vi "Connect TCP.vi"(5 "Connection.TCP in":refnum<class "Connection.TCP.lvclass">, 6 "timeout (100ms)":i32=100, 8 "error in (no error)":errorcluster, 10 "remote port (80)":u16=80, 11 "address (localhost)":string="localhost") -> (0 "error out":errorcluster, 3 "Connection.TCP":refnum<class "Connection.TCP.lvclass">)   [LabVIEW 2013, in "Connection.TCP_GOSPL.lvlib" / "Connection.TCP.lvclass"]
uses:
  Connection.TCP.lvclass
  Connection.TCP.lvclass/Connection.TCP.ctl
  Connection/Connection.lvclass/Connection.ctl
  Connection/Connection.lvclass
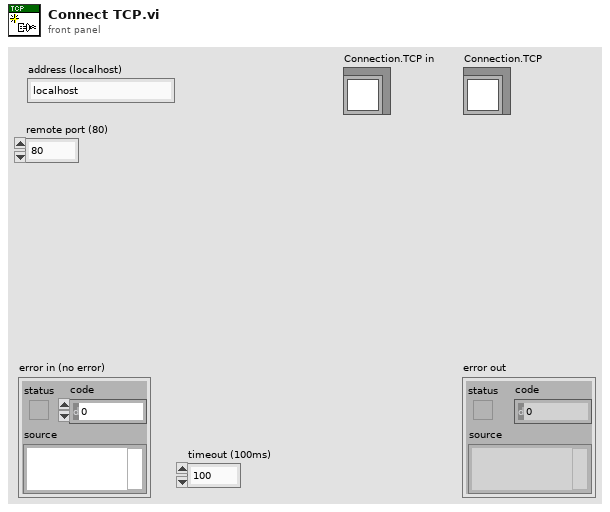
[diagram p1: front panel]
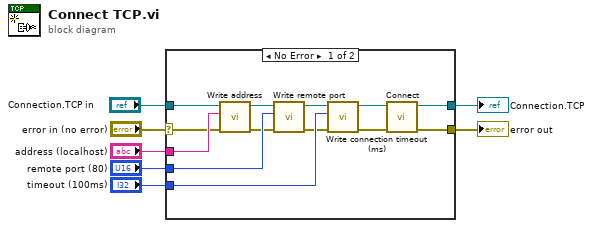
[diagram p0: block diagram]
diagram:
  n1 = case shown="No Error" "error in (no error)" {
    selector: "error in (no error)" -> [w9 w22]
    tunnel: [w19 w22] -> w6
    tunnel: [w20 w21] -> w2
    tunnel: "address (localhost)" -> [w14 _]
    tunnel: "remote port (80)" -> [w12 _]
    tunnel: "timeout (100ms)" -> [w16 _]
    tunnel: "Connection.TCP in" -> [w15 w21]
    frame No Error {
      n2 = call "Write address.vi"("error in (no error)"=w9, "address"=w14, "Connection.TCP"=w15) -> ("error out"=w10:errorcluster, "Connection.TCP"=w13:refnum<class "Connection.TCP.lvclass">)  [unwired: 7 in]
      n3 = call "Write remote port.vi"("error in (no error)"=w10, "remote port (80)"=w12, "Connection.TCP"=w13) -> ("error out"=w8:errorcluster, "Connection.TCP"=w11:refnum<class "Connection.TCP.lvclass">)  [unwired: 7 in]
      n4 = call "Write connection timeout (ms).vi"("error in (no error)"=w8, "connection timeout (ms)"=w16, "Connection in"=w11) -> ("error out"=w17:errorcluster, "Connection out"=w18:refnum<class "Connection.TCP.lvclass">)  [unwired: 7 in]
      n5 = call "Connect.vi"("error in (no error)"=w17, "Connection in"=w18) -> ("error out"=w19:errorcluster, "Connection out"=w20:refnum<class "Connection.TCP.lvclass">)  [unwired: 8 in]
    }
    frame Error {
    }
  }
  "error out" <- w6
  "Connection.TCP" <- w2
